vi "Interface Read to CRLF.vi"(8 "error in":errorcluster, 9 "timeout":i32=10000, 10 "bytes to read":i32, 11 "protocol layer in":refnum<class "Simple Serial Interface.lvclass">) -> (0 "error out":errorcluster, 1 "timed out?":bool, 2 "data":u8[](array[numeric]), 3 "protocol layer out":refnum<class "Simple Serial Interface.lvclass">)   [LabVIEW 2021, in "Simple Serial Interface.lvclass"]
doc: "This provides an interface for reading from a network bus."
uses:
  Simple Serial Interface.lvclass
  Simple Serial Interface.lvclass/Simple Serial Interface.ctl
  Modbus_v121c/Network Interface/Serial Interface/Serial Shared Components/Serial Shared Components.lvlib
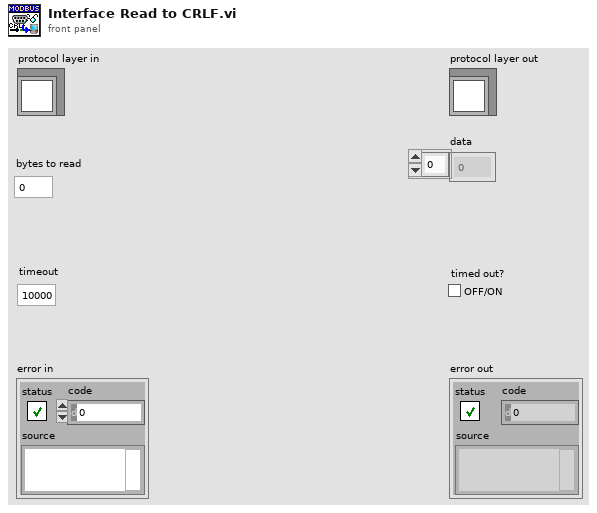
[diagram p1: front panel]
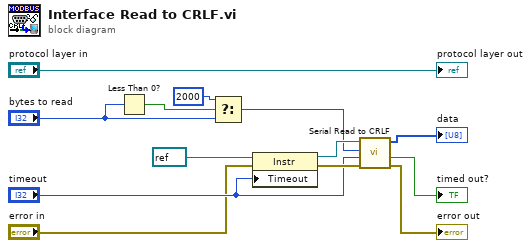
[diagram p0: block diagram]
diagram:
  n1 = Less Than 0?(x="bytes to read") -> (x < 0?=w13:bool)
  n2 = Select(t=u32 2000, s=w13, f="bytes to read") -> (s? t:f=w4:u32)
  n3 = property class="Instr"(reference=refnum<visa-resource-name> refnum, error in="error in", "Timeout"="timeout") -> (reference out=w8:refnum<visa-resource-name>, error out=w10:errorcluster)
  n4 = call "Serial Read to CRLF.vi"("error in"=w10, "timeout (ms)"="timeout", "bytes to read"=w4, "Visa Resource"=w8) -> ("error out"=→"error out":errorcluster, "timed out?"=→"timed out?":bool, "data"=→"data":u8[])  [unwired: 5 in]
  "protocol layer out" <- "protocol layer in"
